vi "AccelerometerSample3.vi"(1 "Period (ms)":u32=5) -> (2 "Ticks":i32, 3 "FIFO full":bool, 4 "Timeouted":bool)   [LabVIEW 2023]
uses:
  <vilib>/rvi/Emulation/niFpgaGetClockAttributes.vi
  <vilib>/rvi/Emulation/niFpgaSctlEmulationGetInTimedLoop.vi
  <vilib>/rvi/Emulation/niFpgaEmulationReportErrorSimple.vi
  <vilib>/rvi/eio/common/nirviEmuTemplateMethod_errors.vi
  <vilib>/rvi/occurrence/nirviWaitOnOccurrenceBase.vi
  <vilib>/rvi/Emulation/niFpgaCriticalErrorInLSC.vi
  <vilib>/rvi/Emulation/niFpgaProcessEmulError.vi
  <vilib>/eio/EIONode/EIONode.xnode
  <vilib>/eio/EIOMethodNode/EIOMethodNode.xnode
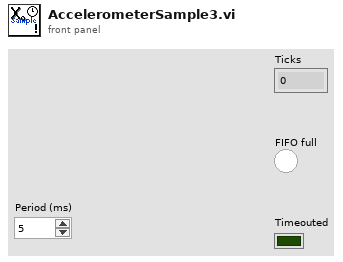
[diagram p1: front panel]
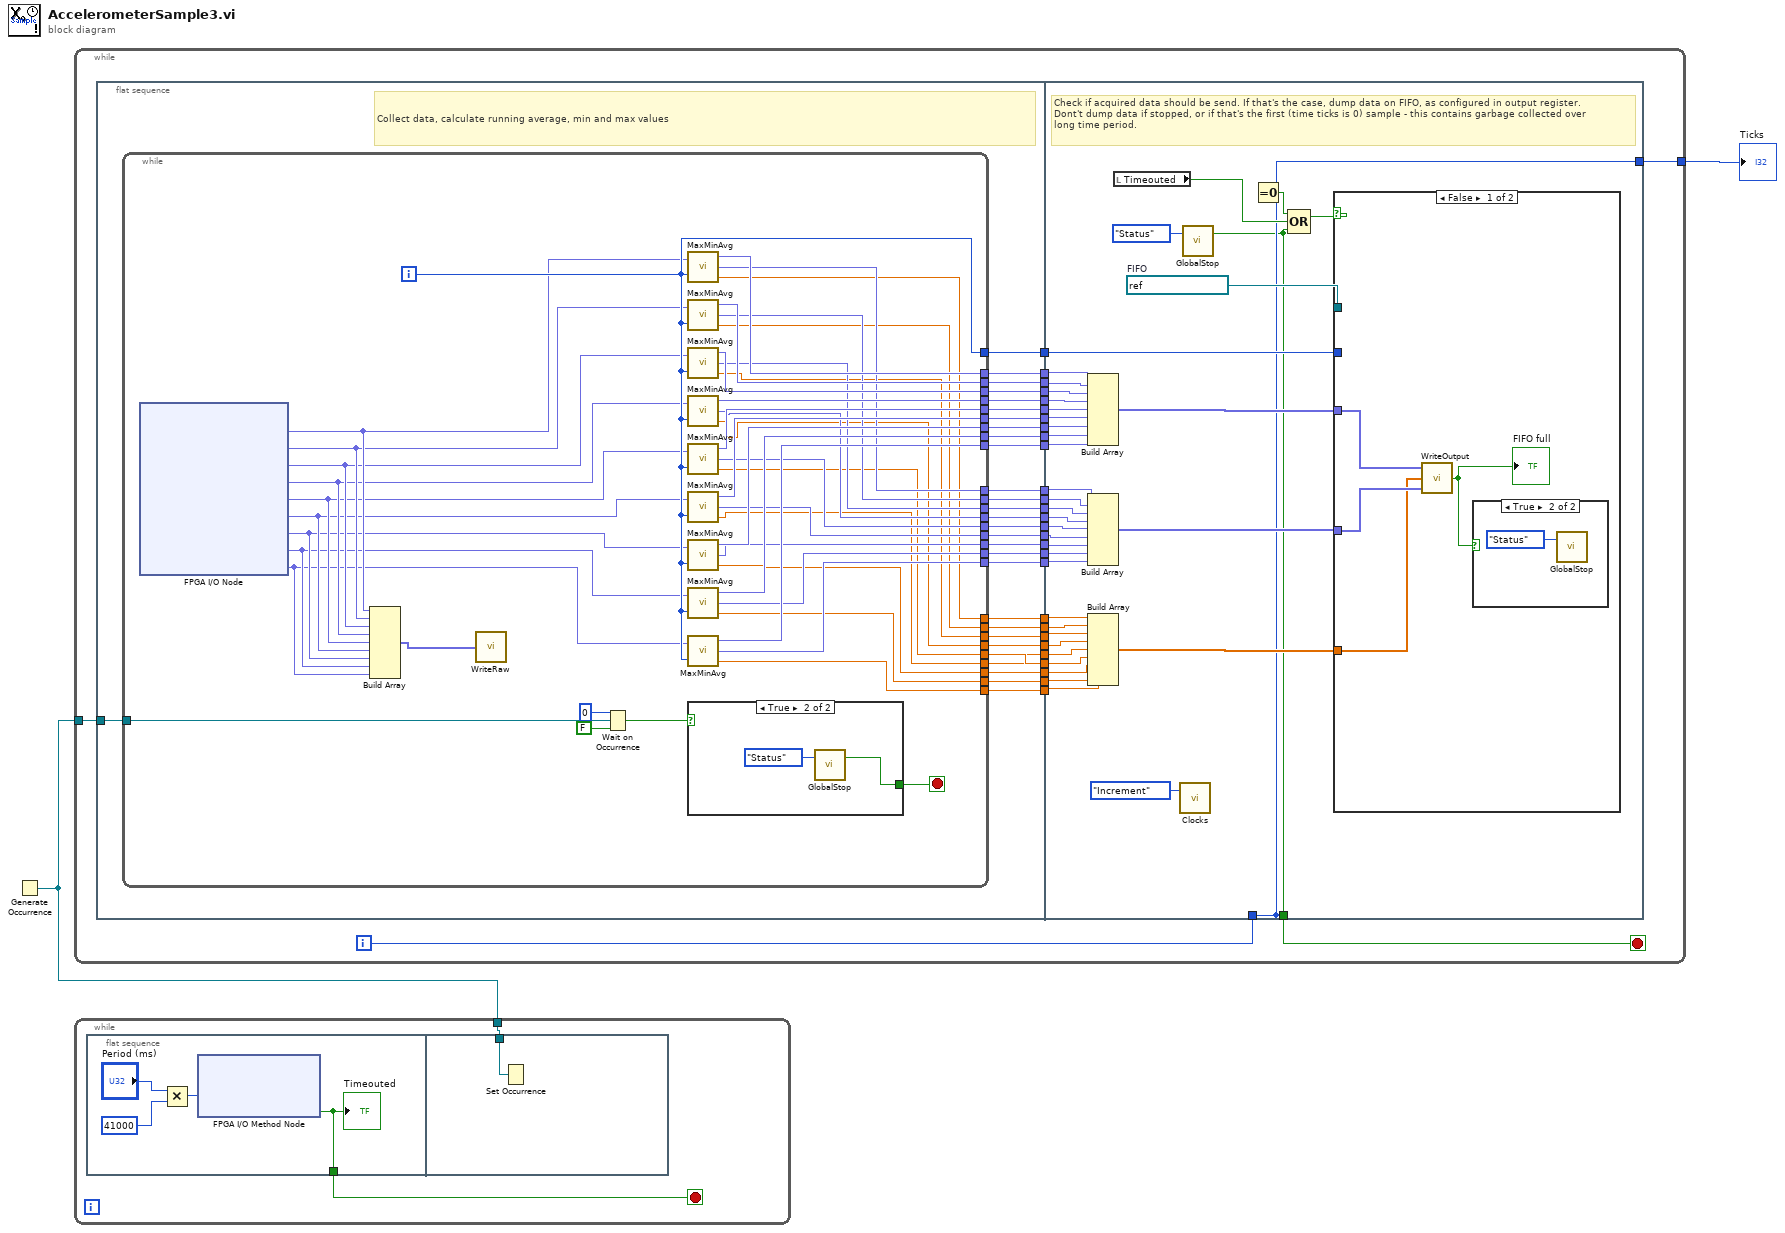
[diagram p0: block diagram]
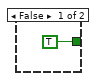
[diagram p2: hidden frame]
diagram:
  n1 = Generate Occurrence() -> (w2:refnum<k4>)
  n2 = while "Sample loop" {
    tunnel: w2 -> [w5]
    tunnel: [w3] -> w1
    i -> [w4]
    stop <- w7 stop-if-true
    n3 = flat-sequence {
      tunnel: [w63] -> w34
      tunnel: [w62] -> w33
      tunnel: [w61] -> w32
      tunnel: [w60] -> w31
      tunnel: [w59] -> w30
      tunnel: [w58] -> w29
      tunnel: [w57] -> w28
      tunnel: [w56] -> w27
      tunnel: [w55] -> w26
      tunnel: [w54] -> w25
      tunnel: [w53] -> w24
      tunnel: [w52] -> w23
      tunnel: [w51] -> w22
      tunnel: [w50] -> w21
      tunnel: [w49] -> w20
      tunnel: [w48] -> w19
      tunnel: [w47] -> w18
      tunnel: [w46] -> w17
      tunnel: [w45] -> w16
      tunnel: [w44] -> w15
      tunnel: [w43] -> w14
      tunnel: [w42] -> w13
      tunnel: [w41] -> w12
      tunnel: [w40] -> w11
      tunnel: [w39] -> w10
      tunnel: [w38] -> w9
      tunnel: [w37] -> w8
      tunnel: [w36] -> w6
      tunnel: w5 -> [w35]
      tunnel: w34 -> [w148]
      tunnel: w33 -> [w147]
      tunnel: w32 -> [w146]
      tunnel: w31 -> [w145]
      tunnel: w30 -> [w144]
      tunnel: w29 -> [w143]
      tunnel: w28 -> [w142]
      tunnel: w27 -> [w141]
      tunnel: w26 -> [w140]
      tunnel: w25 -> [w139]
      tunnel: w24 -> [w138]
      tunnel: w23 -> [w137]
      tunnel: w22 -> [w136]
      tunnel: w21 -> [w135]
      tunnel: w20 -> [w134]
      tunnel: w19 -> [w133]
      tunnel: w18 -> [w132]
      tunnel: w17 -> [w131]
      tunnel: w16 -> [w130]
      tunnel: w15 -> [w129]
      tunnel: w14 -> [w128]
      tunnel: w13 -> [w127]
      tunnel: w12 -> [w122]
      tunnel: w11 -> [w123]
      tunnel: w10 -> [w126]
      tunnel: w9 -> [w125]
      tunnel: w8 -> [w124]
      tunnel: [w111] -> w7
      tunnel: w6 -> [w114]
      tunnel: w4 -> [w113]
      tunnel: [w113] -> _
      tunnel: [w113] -> w3
      frame #0 {
        # "Collect data, calculate running average, min and max values"
        n4 = while {
          tunnel: [w106] -> w63
          tunnel: [w105] -> w62
          tunnel: [w104] -> w61
          tunnel: [w103] -> w60
          tunnel: [w102] -> w59
          tunnel: [w101] -> w58
          tunnel: [w100] -> w57
          tunnel: [w99] -> w56
          tunnel: [w98] -> w55
          tunnel: [w97] -> w54
          tunnel: [w96] -> w53
          tunnel: [w95] -> w52
          tunnel: [w94] -> w51
          tunnel: [w93] -> w50
          tunnel: [w92] -> w49
          tunnel: [w91] -> w48
          tunnel: [w90] -> w47
          tunnel: [w89] -> w46
          tunnel: [w88] -> w45
          tunnel: [w87] -> w44
          tunnel: [w86] -> w43
          tunnel: [w85] -> w42
          tunnel: [w84] -> w41
          tunnel: [w83] -> w40
          tunnel: [w82] -> w39
          tunnel: [w81] -> w38
          tunnel: [w80] -> w37
          tunnel: [w79] -> w36
          tunnel: w35 -> [w76]
          i -> [w79]
          stop <- w78 stop-if-true
          n5 = xnode "FPGA I/O Node"() -> ("Accelerometer1/AI0"=w73:fxp<+/-,24,7>, "Accelerometer1/AI1"=w72:fxp<+/-,24,7>, "Accelerometer1/AI2"=w71:fxp<+/-,24,7>, "Accelerometer2/AI0"=w70:fxp<+/-,24,7>, "Accelerometer2/AI1"=w69:fxp<+/-,24,7>, "Accelerometer2/AI2"=w68:fxp<+/-,24,7>, "Accelerometer3/AI0"=w67:fxp<+/-,24,7>, "Accelerometer3/AI1"=w66:fxp<+/-,24,7>, "Accelerometer3/AI2"=w65:fxp<+/-,24,7>)  [unwired: 9 in, 9 out]
          n6 = Build Array(w73, w72, w71, w70, w69, w68, w67, w66, w65) -> (w64:fxp<+/-,24,7>[])
          n7 = call "WriteRaw.vi"("Array"=w64) -> ()
          n8 = Wait on Occurrence(1:FALSE ("ignore previous (T)"), 2:w76, 3:0 ("ms timeout (-1)")) -> (0:w77:bool)
          n9 = call "MaxMinAvg.vi"("Measurement"=w73, "Index"=w79) -> ("Minimum Value"=w106:fxp<+/-,24,4>, "Maximum Value"=w97:fxp<+/-,24,4>, "Average Value"=w88:sgl)
          n10 = call "MaxMinAvg.vi"("Measurement"=w72, "Index"=w79) -> ("Minimum Value"=w105:fxp<+/-,24,4>, "Maximum Value"=w96:fxp<+/-,24,4>, "Average Value"=w87:sgl)
          n11 = call "MaxMinAvg.vi"("Measurement"=w71, "Index"=w79) -> ("Minimum Value"=w104:fxp<+/-,24,4>, "Maximum Value"=w95:fxp<+/-,24,4>, "Average Value"=w86:sgl)
          n12 = call "MaxMinAvg.vi"("Measurement"=w70, "Index"=w79) -> ("Minimum Value"=w103:fxp<+/-,24,4>, "Maximum Value"=w94:fxp<+/-,24,4>, "Average Value"=w85:sgl)
          n13 = call "MaxMinAvg.vi"("Measurement"=w69, "Index"=w79) -> ("Minimum Value"=w102:fxp<+/-,24,4>, "Maximum Value"=w93:fxp<+/-,24,4>, "Average Value"=w84:sgl)
          n14 = call "MaxMinAvg.vi"("Measurement"=w68, "Index"=w79) -> ("Minimum Value"=w101:fxp<+/-,24,4>, "Maximum Value"=w92:fxp<+/-,24,4>, "Average Value"=w83:sgl)
          n15 = call "MaxMinAvg.vi"("Measurement"=w67, "Index"=w79) -> ("Minimum Value"=w100:fxp<+/-,24,4>, "Maximum Value"=w91:fxp<+/-,24,4>, "Average Value"=w82:sgl)
          n16 = call "MaxMinAvg.vi"("Measurement"=w66, "Index"=w79) -> ("Minimum Value"=w99:fxp<+/-,24,4>, "Maximum Value"=w90:fxp<+/-,24,4>, "Average Value"=w81:sgl)
          n17 = call "MaxMinAvg.vi"("Measurement"=w65, "Index"=w79) -> ("Minimum Value"=w98:fxp<+/-,24,4>, "Maximum Value"=w89:fxp<+/-,24,4>, "Average Value"=w80:sgl)
          n18 = case shown="True" w77 {
            tunnel: [TRUE w108] -> w78
            frame False {
            }
            frame True {
              n19 = call "GlobalStop.vi"("Enum"=enum16{"Clear", "Set", "Status"}."Status") -> ("Boolean"=w108:bool)  [unwired: 1 in, 1 out]
            }
          }
        }
      }
      frame #1 {
        w121 = refnum<k21> "ResponseFIFO"  # FIFO
        # "Check if acquired data should be send. If that's the case, dump data on FIFO, as configured in output register.\nDont't dump data if stopped, or if that's the first (time ticks is 0) sample - this contains garbage collected over\nlong time period."
        n20 = Build Array(w148, w147, w146, w145, w144, w143, w142, w141, w140) -> (w120:fxp<+/-,24,4>[])
        n21 = Build Array(w139, w138, w137, w136, w135, w134, w133, w132, w131) -> (w119:fxp<+/-,24,4>[])
        n22 = Build Array(w130, w129, w128, w127, w123, w122, w126, w125, w124) -> (w118:sgl[])
        n23 = local read "Timeouted"() -> (w115:bool)
        n24 = call "Clocks.vi"("Enum"=enum16{"Reset", "Increment", "Get"}."Increment") -> ()  [unwired: 1 in, 2 out]
        n25 = call "GlobalStop.vi"("Enum"=enum16{"Clear", "Set", "Status"}."Status") -> ("Boolean"=w111:bool)  [unwired: 1 in, 1 out]
        n26 = Equal To 0?(x=w113) -> (x = 0?=w116:bool)
        n27 = Compound Arithmetic op=OR(w116, w115, w111) -> (w117:bool)
        n28 = case shown="False" w117 {
          tunnel: w121 -> [_ _]
          tunnel: w120 -> [w152 _]
          tunnel: w119 -> [w151 _]
          tunnel: w118 -> [w150 _]
          tunnel: w114 -> [_ _]
          frame False {
            n29 = call "WriteOutput.vi"("Max"=w151, "Average"=w150, "Min"=w152) -> ("FIFO full"=w149:bool)
            "FIFO full" <- w149
            n30 = case shown="True" w149 {
              frame False {
              }
              frame True {
                n31 = call "GlobalStop.vi"("Enum"=enum16{"Clear", "Set", "Status"}."Status") -> ()  [unwired: 1 in, 2 out]
              }
            }
          }
          frame True {
          }
        }
      }
    }
  }
  "Ticks" <- w1
  n32 = while {
    tunnel: w2 -> [w154]
    stop <- w155 stop-if-true
    n33 = flat-sequence {
      tunnel: [w156] -> w155
      tunnel: w154 -> [w160]
      frame #0 {
        n34 = Multiply(x="Period (ms)", y=41000) -> (x*y=w158:u32)
        n35 = xnode "FPGA I/O Method Node"("Timeout"=w158) -> ("Timed Out"=w156:bool)  [unwired: 1 in, 1 out]
        "Timeouted" <- w156
      }
      frame #1 {
        n36 = Set Occurrence(w160) -> ()
      }
    }
  }
